vi "Datei im Ordner von VisBx Anzeige.vi"(11 "Dateiname":string="abc") -> (0 "EXE":bool, 2 "Ordner des Haupt-VIs":path, 3 "Dateipfad im Ordner des Haupt-VIs":path)   [LabVIEW 2020, in "Anlagenuebersicht.lvlib" / "VisBx Anzeige.lvlib"]
doc: "Erzeugt einen vollständigen Dateipfad mit dem Namens-Teil \"Dateiname\" und dem Ordner des aktuellen Hauptprogrammes, wenn das Hauptprogramm als Anwendung (.exe) läuft. Für die Entwicklungsphase muss das VI im selben Ordner wie das Haupt-VI liegen."
uses:
  VisBx Anzeige.lvlib
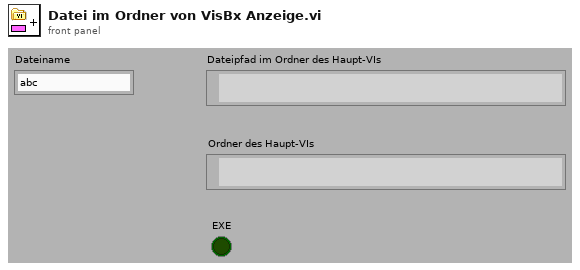
[diagram p1: front panel]
types:
  T1 = enum32{"invalid app kind", "Development System", "Run Time System", "Student Edition", "Embedded LabVIEW", "Evaluation", "Custom"}
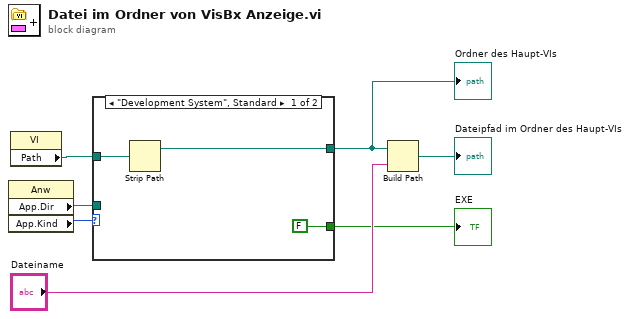
[diagram p0: block diagram]
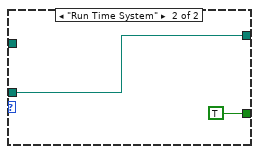
[diagram p2: hidden frame]
diagram:
  n1 = property class="Anw"() -> ("App.Dir"=w3:path, "App.Kind"=w5:T1)  [unwired: 2 in, 2 out]
  n2 = property class="VI"() -> ("Path"=w4:path)  [unwired: 2 in, 2 out]
  n3 = case shown="\"Development System\", Standard" w5 {
    tunnel: w4 -> [w10 _]
    tunnel: w3 -> [_ w12]
    tunnel: [w9 w12] -> w2
    tunnel: [FALSE TRUE] -> w1
    frame "Development System", Default {
      n4 = Strip Path(path=w10) -> (stripped path=w9:path)  [unwired: 1 out]
    }
    frame "Run Time System" {
    }
  }
  "Ordner des Haupt-VIs" <- w2
  "EXE" <- w1
  n5 = Build Path(base path=w2, name or relative path="Dateiname") -> (appended path=→"Dateipfad im Ordner des Haupt-VIs":path)
